vi "Initialize.vi"(8 "error in (no error)":errorcluster, 11 "Instrument in":refnum<class "Instrument.lvclass">) -> (0 "error out":errorcluster, 3 "Instrument out":refnum<class "Instrument.lvclass">)   [LabVIEW 2018, in "Instrument.lvclass"]
uses:
  Instrument.lvclass
  Instrument.lvclass/Instrument.ctl
  Device/Optics/Optics.lvclass/Optics.ctl
  Device/Optics/Opt_Selector/Opt_Selector.lvclass
  C:/Users/devstaff/sparc4/s4gui/Versao ZeroMQ REQ-REP/SPARC4_GUI -v1.0.0 - 20250122_ICS-JSON/Device/Optics/Optics.lvclass
  Device/Optics/Opt_Continuous/Opt_Continuous.lvclass
  Server/Server.lvclass
  Comm/Stream/Stream.lvclass
  Log/Log.lvclass
  StateMachine/State Machine.lvclass
  Device/Optics/Optics.lvclass
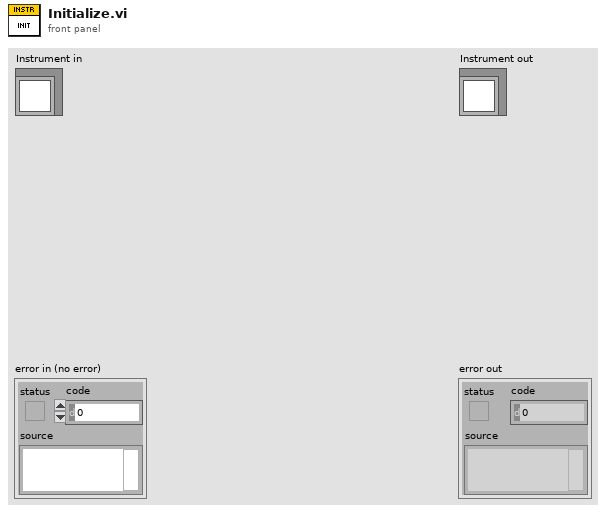
[diagram p1: front panel]
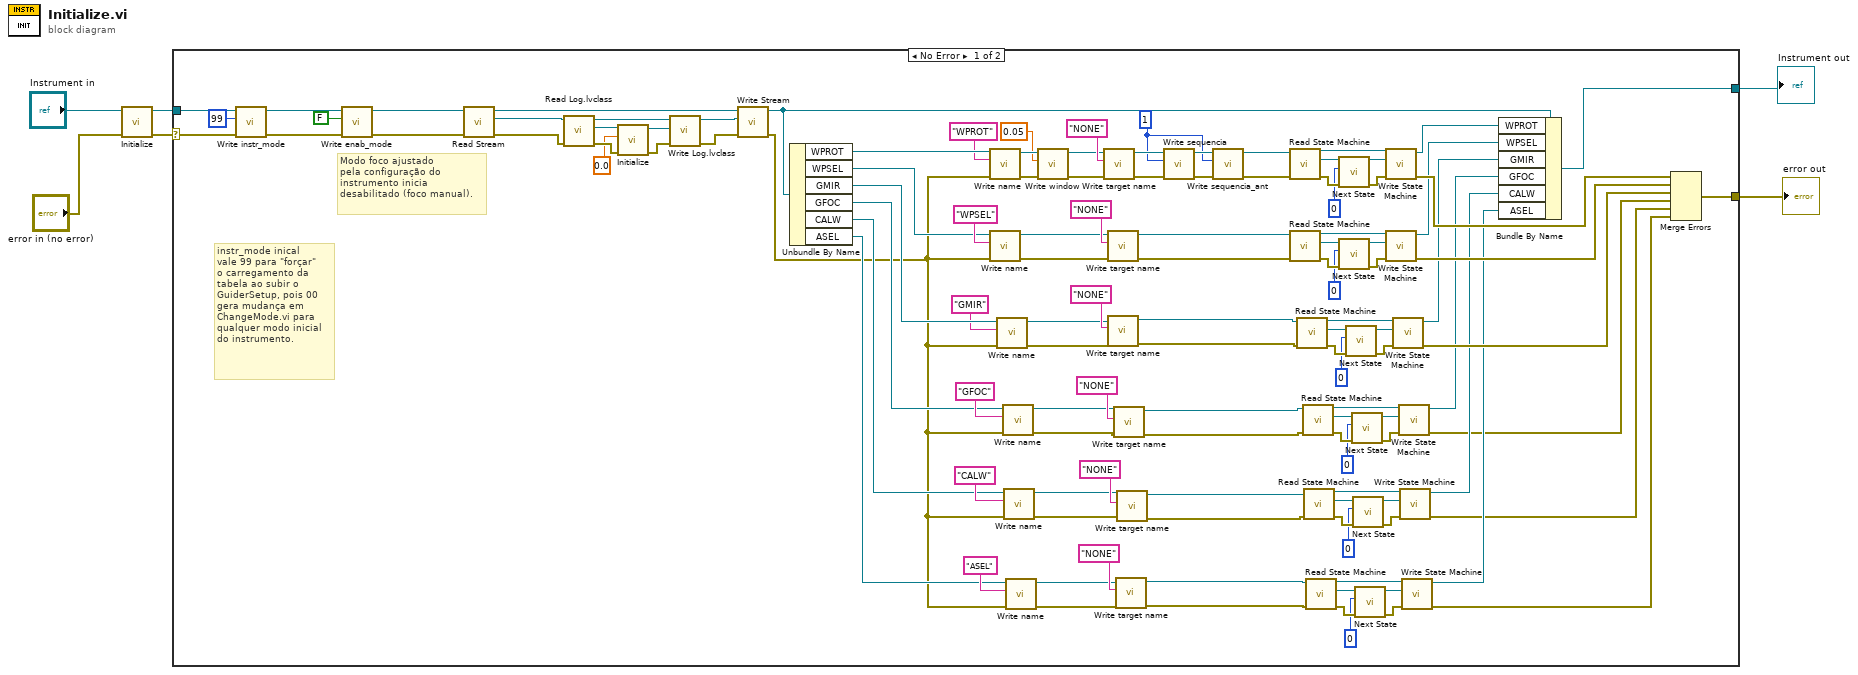
[diagram p0: block diagram]
diagram:
  n1 = call-parent "Initialize.vi"("error in (no error)"="error in (no error)", "Server in"="Instrument in") -> ("error out"=w3:errorcluster, "Server out"=w4:refnum<class "Instrument.lvclass">)  [unwired: 8 in]
  n2 = case shown="No Error" w3 {
    selector: w3 -> [w9 w129]
    tunnel: [w60 w128] -> w1
    tunnel: w4 -> [w11 w128]
    tunnel: [w108 w129] -> w2
    frame No Error {
      w17 = u16 1 ("sequencia")
      # "instr_mode inical \nvale 99 para \"forçar\"\no carregamento da \ntabela ao subir o \nGuiderSetup, pois 00\ngera mudança em\nChangeMode.vi para\nqualquer modo inicial\ndo instrumento."
      # "Modo foco ajustado\npela configuração do\ninstrumento inicia\ndesabilitado (foco manual)."
      n3 = call-dynamic "Write instr_mode.vi"("error in (no error)"=w9, "instr_mode"=u32 99, "Instrument in"=w11) -> ("error out"=w8:errorcluster, "Instrument out"=w10:refnum<class "Instrument.lvclass">)  [unwired: 7 in]
      n4 = call-dynamic "Write enab_mode.vi"("error in (no error)"=w8, "enab_mode"=FALSE, "Instrument in"=w10) -> ("error out"=w12:errorcluster, "Instrument out"=w13:refnum<class "Instrument.lvclass">)  [unwired: 7 in]
      n5 = call-dynamic "Read Stream.vi"("error in (no error)"=w12, "Server in"=w13) -> ("error out"=w14:errorcluster, "Stream.lvclass"=w15:refnum<class "Stream.lvclass">, "Server out"=w127:refnum<class "Instrument.lvclass">)  [unwired: 7 in]
      n6 = call-dynamic "Read Log.lvclass.vi"("error in (no error)"=w14, "Comm in"=w15) -> ("error out"=w28:errorcluster, "Log.lvclass"=w30:refnum<class "Log.lvclass">, "Comm out"=w31:refnum<class "Stream.lvclass">)  [unwired: 7 in]
      n7 = call-dynamic "Initialize.vi"("error in (no error)"=w28, "Level"=0.0, "Log in"=w30) -> ("error out"=w27:errorcluster, "Log out"=w29:refnum<class "Log.lvclass">)  [unwired: 7 in]
      n8 = call-dynamic "Write Log.lvclass.vi"("error in (no error)"=w27, "Log.lvclass"=w29, "Comm in"=w31) -> ("error out"=w25:errorcluster, "Comm out"=w26:refnum<class "Stream.lvclass">)  [unwired: 7 in]
      n9 = call-dynamic "Write Stream.vi"("error in (no error)"=w25, "Stream.lvclass"=w26, "Server in"=w127) -> ("error out"=w70:errorcluster, "Server out"=w61:refnum<class "Instrument.lvclass">)  [unwired: 7 in]
      n10 = Unbundle By Name(w61) -> ("WPROT"=w119:refnum<class "Opt_Selector.lvclass">, "WPSEL"=w110:refnum<class "Opt_Selector.lvclass">, "GMIR"=w99:refnum<class "Opt_Continuous.lvclass">, "GFOC"=w88:refnum<class "Opt_Continuous.lvclass">, "CALW"=w72:refnum<class "Opt_Selector.lvclass">, "ASEL"=w71:refnum<class "Opt_Selector.lvclass">)
      n11 = call-dynamic "Write name.vi"("error in (no error)"=w70, "name"="WPROT", "Optics in"=w119) -> ("error out"=w64:errorcluster, "Optics out"=w63:refnum<class "Opt_Selector.lvclass">)  [unwired: 7 in]
      n12 = call-dynamic "Write name.vi"("error in (no error)"=w70, "name"="WPSEL", "Optics in"=w110) -> ("error out"=w54:errorcluster, "Optics out"=w55:refnum<class "Opt_Selector.lvclass">)  [unwired: 7 in]
      n13 = call-dynamic "Write name.vi"("error in (no error)"=w70, "name"="GMIR", "Optics in"=w99) -> ("error out"=w45:errorcluster, "Optics out"=w47:refnum<class "Opt_Continuous.lvclass">)  [unwired: 7 in]
      n14 = call-dynamic "Write name.vi"("error in (no error)"=w70, "name"="GFOC", "Optics in"=w88) -> ("error out"=w41:errorcluster, "Optics out"=w43:refnum<class "Opt_Continuous.lvclass">)  [unwired: 7 in]
      n15 = call-dynamic "Write name.vi"("error in (no error)"=w70, "name"="CALW", "Optics in"=w72) -> ("error out"=w37:errorcluster, "Optics out"=w39:refnum<class "Opt_Selector.lvclass">)  [unwired: 7 in]
      n16 = call-dynamic "Write name.vi"("error in (no error)"=w70, "name"="ASEL", "Optics in"=w71) -> ("error out"=w33:errorcluster, "Optics out"=w35:refnum<class "Opt_Selector.lvclass">)  [unwired: 7 in]
      n17 = call "Write window.vi"("error in (no error)"=w64, "window"=0.05, "Optics in"=w63) -> ("error out"=w57:errorcluster, "Optics out"=w58:refnum<class "Opt_Selector.lvclass">)  [unwired: 7 in]
      n18 = call "Write target name.vi"("error in (no error)"=w57, "target name"="NONE", "Optics in"=w58) -> ("error out"=w20:errorcluster, "Optics out"=w23:refnum<class "Opt_Selector.lvclass">)  [unwired: 7 in]
      n19 = call "Write target name.vi"("error in (no error)"=w54, "target name"="NONE", "Optics in"=w55) -> ("error out"=w53:errorcluster, "Optics out"=w52:refnum<class "Opt_Selector.lvclass">)  [unwired: 7 in]
      n20 = call "Write target name.vi"("error in (no error)"=w45, "target name"="NONE", "Optics in"=w47) -> ("error out"=w44:errorcluster, "Optics out"=w46:refnum<class "Opt_Continuous.lvclass">)  [unwired: 7 in]
      n21 = call "Write target name.vi"("error in (no error)"=w41, "target name"="NONE", "Optics in"=w43) -> ("error out"=w40:errorcluster, "Optics out"=w42:refnum<class "Opt_Continuous.lvclass">)  [unwired: 7 in]
      n22 = call "Write target name.vi"("error in (no error)"=w33, "target name"="NONE", "Optics in"=w35) -> ("error out"=w32:errorcluster, "Optics out"=w34:refnum<class "Opt_Selector.lvclass">)  [unwired: 7 in]
      n23 = call "Write target name.vi"("error in (no error)"=w37, "target name"="NONE", "Optics in"=w39) -> ("error out"=w36:errorcluster, "Optics out"=w38:refnum<class "Opt_Selector.lvclass">)  [unwired: 7 in]
      n24 = call-dynamic "Write sequencia.vi"("error in (no error)"=w20, "sequencia"=w17, "Opt_Selector in"=w23) -> ("error out"=w19:errorcluster, "Opt_Selector out"=w22:refnum<class "Opt_Selector.lvclass">)  [unwired: 7 in]
      n25 = call-dynamic "Write sequencia_ant.vi"("error in (no error)"=w19, "sequencia_ant"=w17, "Opt_Selector in"=w22) -> ("error out"=w18:errorcluster, "Opt_Selector out"=w21:refnum<class "Opt_Selector.lvclass">)  [unwired: 7 in]
      n26 = call-dynamic "Read State Machine.vi"("error in (no error)"=w18, "Device in"=w21) -> ("error out"=w123:errorcluster, "State Machine.lvclass"=w126:refnum<class "State Machine.lvclass">, "Device out"=w125:refnum<class "Opt_Selector.lvclass">)  [unwired: 7 in]
      n27 = call-dynamic "Read State Machine.vi"("error in (no error)"=w53, "Device in"=w52) -> ("error out"=w114:errorcluster, "State Machine.lvclass"=w117:refnum<class "State Machine.lvclass">, "Device out"=w116:refnum<class "Opt_Selector.lvclass">)  [unwired: 7 in]
      n28 = call-dynamic "Read State Machine.vi"("error in (no error)"=w44, "Device in"=w46) -> ("error out"=w102:errorcluster, "State Machine.lvclass"=w105:refnum<class "State Machine.lvclass">, "Device out"=w104:refnum<class "Opt_Continuous.lvclass">)  [unwired: 7 in]
      n29 = call-dynamic "Read State Machine.vi"("error in (no error)"=w40, "Device in"=w42) -> ("error out"=w92:errorcluster, "State Machine.lvclass"=w95:refnum<class "State Machine.lvclass">, "Device out"=w94:refnum<class "Opt_Continuous.lvclass">)  [unwired: 7 in]
      n30 = call-dynamic "Read State Machine.vi"("error in (no error)"=w36, "Device in"=w38) -> ("error out"=w83:errorcluster, "State Machine.lvclass"=w86:refnum<class "State Machine.lvclass">, "Device out"=w85:refnum<class "Opt_Selector.lvclass">)  [unwired: 7 in]
      n31 = call-dynamic "Read State Machine.vi"("error in (no error)"=w32, "Device in"=w34) -> ("error out"=w76:errorcluster, "State Machine.lvclass"=w79:refnum<class "State Machine.lvclass">, "Device out"=w78:refnum<class "Opt_Selector.lvclass">)  [unwired: 7 in]
      n32 = call "Next State.vi"("error in (no error)"=w123, "New_State"=0, "State Machine in"=w126) -> ("error out"=w122:errorcluster, "State Machine out"=w124:refnum<class "State Machine.lvclass">)  [unwired: 7 in]
      n33 = call "Next State.vi"("error in (no error)"=w114, "New_State"=0, "State Machine in"=w117) -> ("error out"=w113:errorcluster, "State Machine out"=w115:refnum<class "State Machine.lvclass">)  [unwired: 7 in]
      n34 = call "Next State.vi"("error in (no error)"=w102, "New_State"=0, "State Machine in"=w105) -> ("error out"=w101:errorcluster, "State Machine out"=w103:refnum<class "State Machine.lvclass">)  [unwired: 7 in]
      n35 = call "Next State.vi"("error in (no error)"=w92, "New_State"=0, "State Machine in"=w95) -> ("error out"=w91:errorcluster, "State Machine out"=w93:refnum<class "State Machine.lvclass">)  [unwired: 7 in]
      n36 = call "Next State.vi"("error in (no error)"=w83, "New_State"=0, "State Machine in"=w86) -> ("error out"=w82:errorcluster, "State Machine out"=w84:refnum<class "State Machine.lvclass">)  [unwired: 7 in]
      n37 = call "Next State.vi"("error in (no error)"=w76, "New_State"=0, "State Machine in"=w79) -> ("error out"=w75:errorcluster, "State Machine out"=w77:refnum<class "State Machine.lvclass">)  [unwired: 7 in]
      n38 = call-dynamic "Write State Machine.vi"("error in (no error)"=w122, "State Machine.lvclass"=w124, "Device in"=w125) -> ("error out"=w109:errorcluster, "Device out"=w120:refnum<class "Opt_Selector.lvclass">)  [unwired: 7 in]
      n39 = call-dynamic "Write State Machine.vi"("error in (no error)"=w113, "State Machine.lvclass"=w115, "Device in"=w116) -> ("error out"=w107:errorcluster, "Device out"=w106:refnum<class "Opt_Selector.lvclass">)  [unwired: 7 in]
      n40 = call-dynamic "Write State Machine.vi"("error in (no error)"=w101, "State Machine.lvclass"=w103, "Device in"=w104) -> ("error out"=w97:errorcluster, "Device out"=w98:refnum<class "Opt_Continuous.lvclass">)  [unwired: 7 in]
      n41 = call-dynamic "Write State Machine.vi"("error in (no error)"=w91, "State Machine.lvclass"=w93, "Device in"=w94) -> ("error out"=w65:errorcluster, "Device out"=w87:refnum<class "Opt_Continuous.lvclass">)  [unwired: 7 in]
      n42 = call-dynamic "Write State Machine.vi"("error in (no error)"=w82, "State Machine.lvclass"=w84, "Device in"=w85) -> ("error out"=w67:errorcluster, "Device out"=w69:refnum<class "Opt_Selector.lvclass">)  [unwired: 7 in]
      n43 = call-dynamic "Write State Machine.vi"("error in (no error)"=w75, "State Machine.lvclass"=w77, "Device in"=w78) -> ("error out"=w66:errorcluster, "Device out"=w68:refnum<class "Opt_Selector.lvclass">)  [unwired: 7 in]
      n44 = Bundle By Name(cluster=w61, "WPROT"=w120, "WPSEL"=w106, "GMIR"=w98, "GFOC"=w87, "CALW"=w69, "ASEL"=w68) -> (w60:refnum<class "Instrument.lvclass">)
      n45 = Merge Errors(w109, w107, w97, w65, w67, w66) -> (w108:errorcluster)
    }
    frame Error {
    }
  }
  "error out" <- w2
  "Instrument out" <- w1
